vi "Example3-Inheritance.vi"() -> ()   [LabVIEW 2021]
doc: "Example of object inheritance properties in LabVIEW. Comments in Polish."
uses:
  Spaceship/Spaceship.lvclass
  X-wing/X-wing.lvclass
  Hyperspace_SpaceShip/Hyperspace_SpaceShip.lvclass
  Droid/Droid.lvclass
  Astromech droid/Astromech droid.lvclass
panel:
  out "Generic Class":refnum<class "Spaceship.lvclass">
  out "Class Name":string
  out "Error Out 2":errorcluster
  out "Class Paths Array":path[](array[path])
  out "Specific Class":refnum<class "X-wing.lvclass">
  out "Error Out":errorcluster
  out "Class Name 2":string
  out "appended array":refnum<class "Spaceship.lvclass">[](array[class])
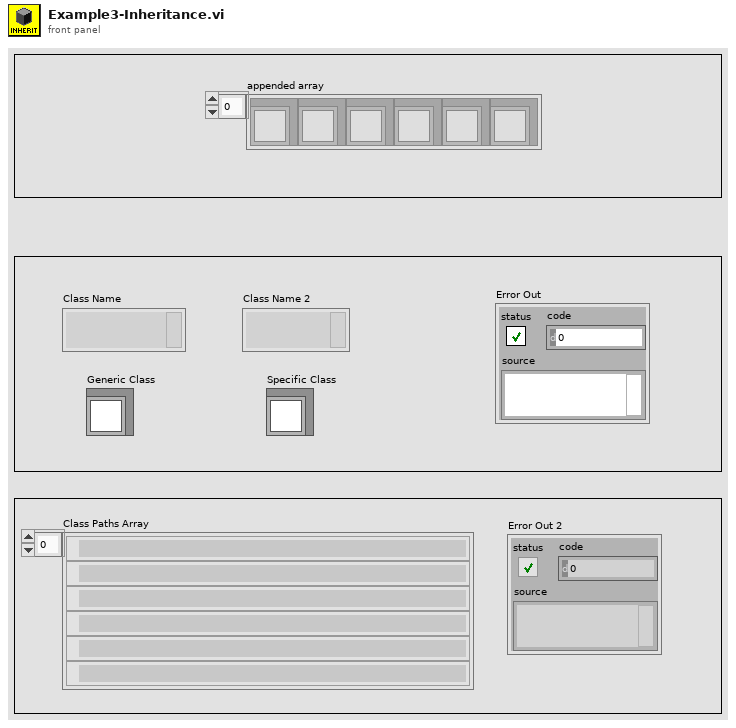
[diagram p1: front panel]
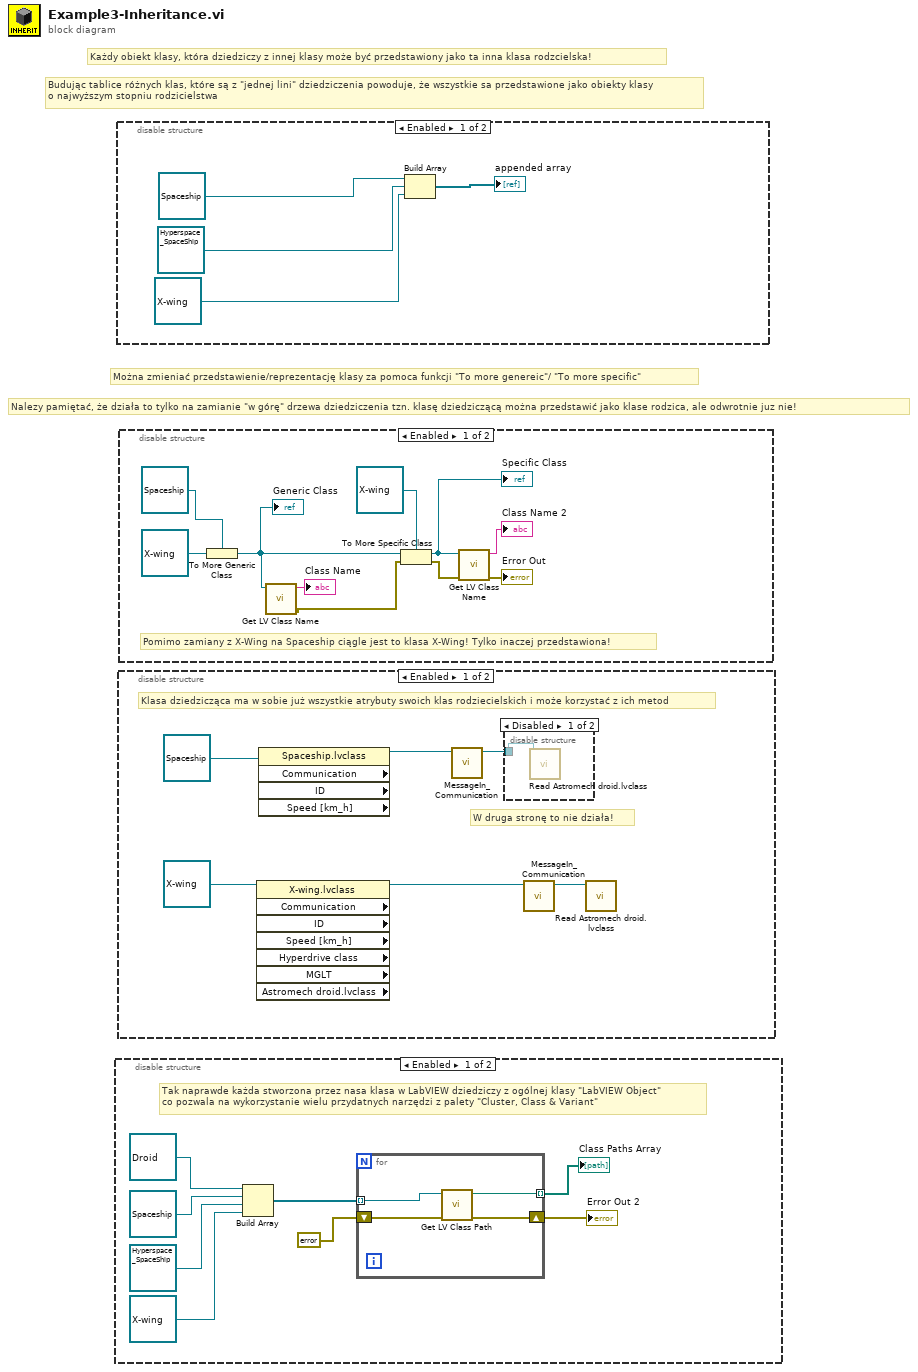
[diagram p0: block diagram]
diagram:
  # "Nalezy pamiętać, że działa to tylko na zamianie \"w górę\" drzewa dziedziczenia tzn. klasę dziedziczącą można przedstawić jako klase rodzica, ale odwrotnie juz nie!"
  # "Można zmieniać przedstawienie/reprezentację klasy za pomoca funkcji \"To more genereic\"/ \"To more specific\""
  # "Każdy obiekt klasy, która dziedziczy z innej klasy może być przedstawiony jako ta inna klasa rodzcielska!"
  # "Budując tablice różnych klas, które są z \"jednej lini\" dziedziczenia powoduje, że wszystkie sa przedstawione jako obiekty klasy\no najwyższym stopniu rodzicielstwa"
  n1 = disable-structure shown="Enabled" {
    frame Enabled {
      # "Tak naprawde każda stworzona przez nasa klasa w LabVIEW dziedziczy z ogólnej klasy \"LabVIEW Object\"\nco pozwala na wykorzystanie wielu przydatnych narzędzi z palety \"Cluster, Class & Variant\""
      n2 = Build Array(refnum<class "Droid.lvclass"> refnum ("Droid.lvclass"), refnum<class "Spaceship.lvclass"> refnum ("Spaceship.lvclass"), refnum<class "Hyperspace_SpaceShip.lvclass"> refnum ("Hyperspace_SpaceShip.lvclass"), refnum<class "X-wing.lvclass"> refnum ("X-wing.lvclass")) -> (w4:refnum<class>[])
      n3 = for {
        tunnel: w4 -> [w12] mode=indexing
        tunnel: [w11] -> w3 mode=indexing
        shift-right: [w10] -> w1
        shift-left: errorcluster {"status"=FALSE, "code"=0, "source"=""} ("error out") -> [w9]
        n4 = call <vilib>:"Get LV Class Path.vi"("error in (no error)"=w9, "object"=w12) -> ("error out"=w10:errorcluster, "class path"=w11:path)  [unwired: 8 in]
      }
      "Class Paths Array" <- w3
      "Error Out 2" <- w1
    }
    frame Disabled {
    }
  }
  n5 = disable-structure shown="Enabled" {
    frame Enabled {
      n6 = Build Array(refnum<class "Spaceship.lvclass"> refnum ("Spaceship.lvclass"), refnum<class "Hyperspace_SpaceShip.lvclass"> refnum ("Hyperspace_SpaceShip.lvclass"), refnum<class "X-wing.lvclass"> refnum ("X-wing.lvclass")) -> (→"appended array":refnum<class "Spaceship.lvclass">[])
    }
    frame Disabled {
    }
  }
  n7 = disable-structure shown="Enabled" {
    frame Enabled {
      # "W druga stronę to nie działa!"
      # "Klasa dziedzicząca ma w sobie już wszystkie atrybuty swoich klas rodziecielskich i może korzystać z ich metod"
      n8 = property class="X-wing.lvclass" props=["Communication", "ID", "Speed [km_h]", "Hyperdrive class", "MGLT", "Astromech droid.lvclass"](reference=refnum<class "X-wing.lvclass"> refnum ("X-wing.lvclass")) -> (reference out=w19:refnum<class "X-wing.lvclass">)  [unwired: 1 in, 7 out]
      n9 = property class="Spaceship.lvclass" props=["Communication", "ID", "Speed [km_h]"](reference=refnum<class "Spaceship.lvclass"> refnum ("Spaceship.lvclass")) -> (reference out=w20:refnum<class "Spaceship.lvclass">)  [unwired: 1 in, 4 out]
      n10 = call-dynamic "MessageIn_Communication.vi"("Spaceship in"=w20) -> ("Spaceship out"=w17:refnum<class "Spaceship.lvclass">)  [unwired: 9 in, 1 out]
      n11 = disable-structure shown="Disabled" {
        disable-tunnel: w17 -> [w23 _]
        frame Disabled {
          n12 = call-dynamic "Read Astromech droid.lvclass.vi"("X-wing in"=w23) -> ()  [unwired: 8 in, 3 out]
        }
        frame Enabled {
        }
      }
      n13 = call-dynamic "MessageIn_Communication.vi"("Spaceship in"=w19) -> ("Spaceship out"=w18:refnum<class "X-wing.lvclass">)  [unwired: 9 in, 1 out]
      n14 = call-dynamic "Read Astromech droid.lvclass.vi"("X-wing in"=w18) -> ()  [unwired: 8 in, 3 out]
    }
    frame Disabled {
    }
  }
  n15 = disable-structure shown="Enabled" {
    frame Enabled {
      # "Pomimo zamiany z X-Wing na Spaceship ciągle jest to klasa X-Wing! Tylko inaczej przedstawiona!"
      n16 = To More Generic Class(target class=refnum<class "Spaceship.lvclass"> refnum ("Spaceship.lvclass"), reference=refnum<class "X-wing.lvclass"> refnum ("X-wing.lvclass")) -> (generic class reference=w26:refnum<class "Spaceship.lvclass">)
      "Generic Class" <- w26
      n17 = call <vilib>:"Get LV Class Name.vi"("object"=w26) -> ("error out"=w25:errorcluster, "class name"=→"Class Name":string)  [unwired: 9 in]
      n18 = To More Specific Class(target class=refnum<class "X-wing.lvclass"> refnum ("X-wing.lvclass"), reference=w26, error in=w25) -> (specific class reference=w31:refnum<class "X-wing.lvclass">, error out=w24:errorcluster)
      "Specific Class" <- w31
      n19 = call <vilib>:"Get LV Class Name.vi"("error in (no error)"=w24, "object"=w31) -> ("error out"=→"Error Out":errorcluster, "class name"=→"Class Name 2":string)  [unwired: 8 in]
    }
    frame Disabled {
    }
  }
